vi "Set Function Generator Parameters SP.vi"(8 "error in":errorcluster, 10 "Function Generator":T1) -> (0 "error out":errorcluster)   [LabVIEW 2025, in "Power Supply.lvlib"]
doc: "Sets the function generator parametrrs setpoint.\n\n_____\nCreated using DQMH Framework: Event Scripter 7.1.1.1528."
uses:
  Power Supply.lvlib
  Function Generator Parameters--cluster.ctl
  Set Function Generator Parameters SP Argument--cluster.ctl
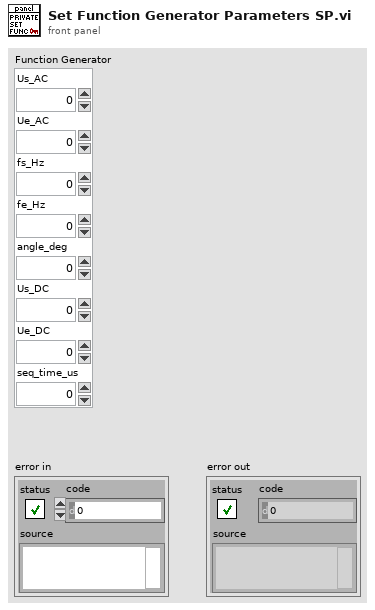
[diagram p1: front panel]
types:
  T1 = typedef "Power Supply.lvlib/Function Generator Parameters--cluster.ctl" = cluster{"Us_AC":sgl, "Ue_AC":sgl, "fs_Hz":sgl, "fe_Hz ":sgl, "angle_deg ":sgl, "Us_DC ":sgl, "Ue_DC":sgl, "seq_time_us":sgl}
  T2 = typedef "Power Supply.lvlib/Set Function Generator Parameters SP Argument--cluster.ctl" = cluster{"Function Generator":T1}
  T3 = typedef "Power Supply.lvlib/Request Events--cluster.ctl" = cluster{"Stop Module":refnum<user-event>, "Show Panel":refnum<user-event>, "Hide Panel":refnum<user-event>, "Get Module Execution Status":refnum<user-event>, "Show Diagram":refnum<user-event>, "Change Panel":refnum<user-event>, "Set Current SP":refnum<user-event>, "Set Voltage SP":refnum<user-event>, "Set Power SP":refnum<user-event>, "Set Power Supply Plugin":refnum<user-event>, "Set DC Output":refnum<user-event>, "Private":cluster{"Sleep Connection Helper Loop":refnum<user-event>}, "Connect":refnum<user-event>, "Disconnect":refnum<user-event>, "Set Function Generator State":refnum<user-event>, "Private.Wake Connection Helper Loop":refnum<user-event>, "Private.Set DC Current SP":refnum<user-event>, "Private.Set DC Voltage SP":refnum<user-event>, "Private.Set DC Power SP":refnum<user-event>, "Private.Set DC Output SP":refnum<user-event>, "Set Function Generator Parameters":refnum<user-event>, "Private.Set Function Generator Parameters SP":refnum<user-event>, "Private.Set Function Generator State SP":refnum<user-event>}
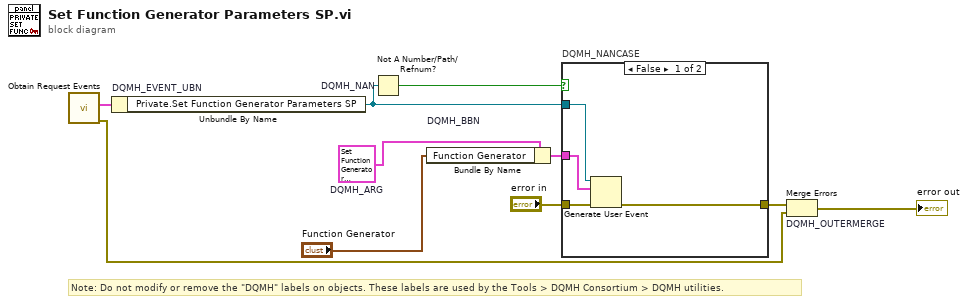
[diagram p0: block diagram]
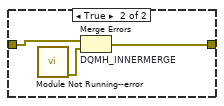
[diagram p2: hidden frame]
diagram:
  w4 = T2 {"Function Generator"={"Us_AC"=0.0, "Ue_AC"=0.0, "fs_Hz"=0.0, "fe_Hz "=0.0, "angle_deg "=0.0, "Us_DC "=0.0, "Ue_DC"=0.0, "seq_time_us"=0.0}}  # DQMH_ARG
  # "Note: Do not modify or remove the \"DQMH\" labels on objects. These labels are used by the Tools > DQMH Consortium > DQMH utilities."
  n1 = call "Obtain Request Events.vi"() -> ("error out"=w2:errorcluster, "Power Supply Request Events"=w1:T3)  [unwired: 10 in]
  n2 = Unbundle By Name "DQMH_EVENT_UBN"(w1) -> ("Private.Set Function Generator Parameters SP"=w6:refnum<user-event>)
  n3 = Not A Number/Path/Refnum? "DQMH_NAN"(number/path/refnum=w6) -> (NaN/Path/Refnum?=w7:bool)
  n4 = Bundle By Name "DQMH_BBN"(cluster=w4, "Function Generator"="Function Generator") -> (w8:T2)
  n5 = case "DQMH_NANCASE" shown="False" w7 {
    tunnel: "error in" -> [w14 w17]
    tunnel: [w13 w16] -> w5
    tunnel: w6 -> [w12 _]
    tunnel: w8 -> [w11 _]
    frame False {
      n6 = Generate User Event(user event=w12, event data cluster=w11, error in=w14) -> (error out=w13:errorcluster)  [unwired: 1 in, 1 out]
    }
    frame True {
      n7 = call "Module Not Running--error.vi"() -> ("error out"=w15:errorcluster)  [unwired: 11 in]
      n8 = Merge Errors "DQMH_INNERMERGE"(w17, w15) -> (w16:errorcluster)
    }
  }
  n9 = Merge Errors "DQMH_OUTERMERGE"(w5, w2) -> (→"error out":errorcluster)
